vi "Setup subWorker - AppMgr.vi"(8 "error in":errorcluster, 11 "Debug Server in":refnum<class "Debug Server.lvclass">) -> (0 "error out":errorcluster, 3 "Debug Server out":refnum<class "Debug Server.lvclass">)   [LabVIEW 2017, in "Debug Server.lvclass"]
doc: "<b>Note: Do not change the code in this VI!</b>\nThis VI performs a setup of all the statically-linked subWorkers that belong to the Worker that calls this VI. This VI is created automatically by the 'Create/Add Worker' tool and must be called <b>before</b> any statically linked subWorkers are called."
uses:
  Debug Server.lvclass
  Debug Server.lvclass/Debug Server.ctl
  Application Manager/Application Manager.lvclass
  C:/Program Files (x86)/National Instruments/LabVIEW 2017/vi.lib/addons/_Workers/Library/Classes/Worker/Worker.lvclass
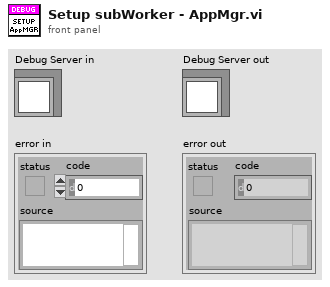
[diagram p1: front panel]
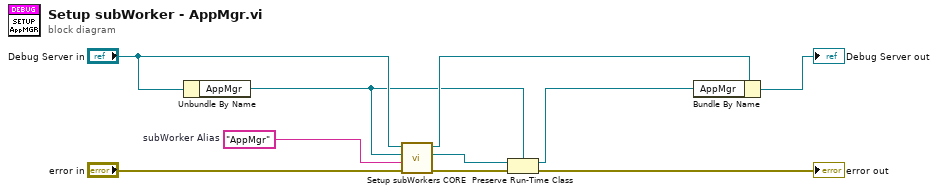
[diagram p0: block diagram]
diagram:
  w6 = "AppMgr"  # subWorker Alias
  n1 = Unbundle By Name("Debug Server in") -> ("AppMgr"=w3:refnum<class "Application Manager.lvclass">)
  n2 = call-dynamic "Setup subWorkers CORE.vi"("error in"="error in", "subWorker Alias"=w6, "subWorker"=w3, "Worker"="Debug Server in") -> ("error out"=w5:errorcluster, "subWorker out"=w1:refnum<class "Worker.lvclass">, "Worker out"=w8:refnum<class "Debug Server.lvclass">)  [unwired: 5 in]
  n3 = Preserve Run-Time Class(object in=w1, error in=w5, 2:w3) -> (object out=w2:refnum<class "Application Manager.lvclass">, error out=→"error out":errorcluster)
  n4 = Bundle By Name(cluster=w8, "AppMgr"=w2) -> (→"Debug Server out":refnum<class "Debug Server.lvclass">)
